vi "Apply Theme To TitleBar-Title.vi"(8 "Error In":errorcluster, 9 "Override Root With (Empty)":string, 10 "Title Ref":refnum<vi>, 11 "ini Theme in":refnum<class "ini Theme.lvclass">) -> (0 "Error Out":errorcluster, 3 "ini Theme out":refnum<class "ini Theme.lvclass">)   [LabVIEW 2021, in "Appearance Actor.lvlib" / "ini Theme.lvclass"]
uses:
  ini Theme.lvclass
  Generic Theme/API/Typedefs/Theme Entry--enum.ctl
  ini Theme.lvclass/ini Theme.ctl
  fa3b262b-9dee-4a2a-a40e-e8b24c2842d1.vi
  e580e7d3-37e0-4797-b7d4-6ea3cff1905c.vi
  b8bb2fda-9813-45b3-b864-ea548737c1bf.vi
  b36eaa81-33c9-40cb-a7ae-b56a33b86463.vi
  de97227f-fe4a-4e4e-bc85-f47ccb7673e6.vi
  5e2e6f35-8fd1-4567-afd0-e7bdc9ba1b23.vi
  7a2ed2a5-f796-4ddb-af4e-0a1f18797397.vi
  c737fe2c-22ae-4e1e-9e67-9ef794ffab69.vi
  <vilib>/Utility/config.llb/Read Key (U32).vi
  <vilib>/Utility/config.llb/Read Key (String).vi
  <vilib>/Utility/config.llb/NI_LVConfig.lvlib
  Generic Theme/Generic Theme.lvclass
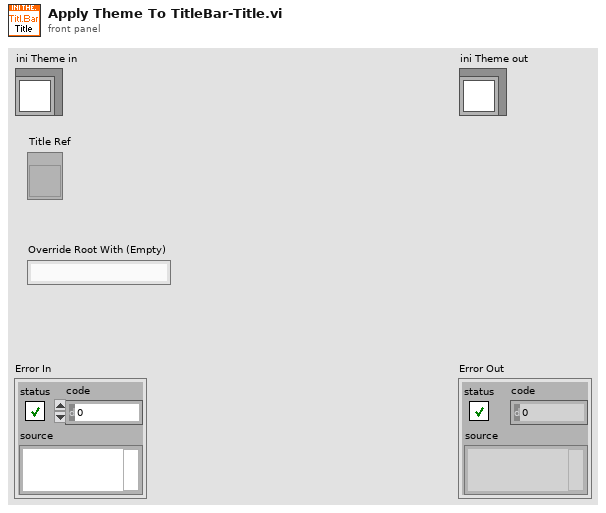
[diagram p1: front panel]
types:
  T1 = typedef "Appearance Actor.lvlib/Generic Theme.lvclass/Theme Entry--enum.ctl" = enum16{"None", "TitleBar.Pane.Color", "TitleBar.Splitter.FillColor", "TitleBar.Splitter.OutlineColor", "TitleBar.Title.Font.Color", "TitleBar.Title.Font.Family", "TitleBar.Title.Font.Size", "TitleBar.Title.Font.Style"}
  T2 = typedef "NI_LVConfig.lvlib/Config Data RefNum.ctl" = refnum<k1>
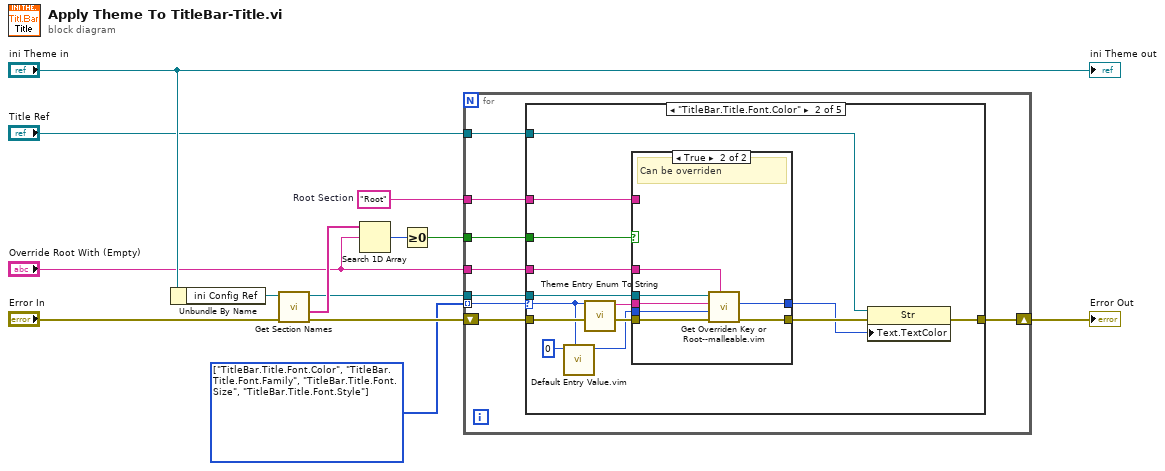
[diagram p0: block diagram]
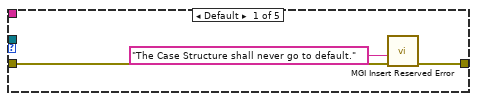
[diagram p2: hidden frame]
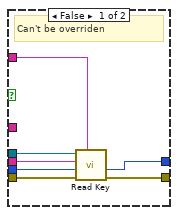
[diagram p3: hidden frame]
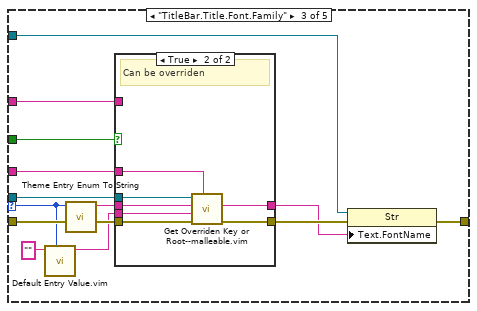
[diagram p4: hidden frame]
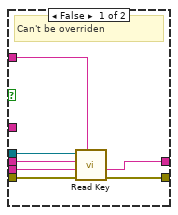
[diagram p5: hidden frame]
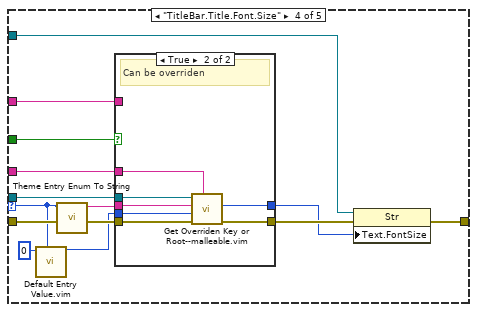
[diagram p6: hidden frame]
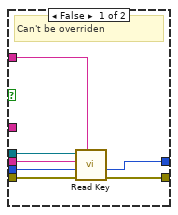
[diagram p7: hidden frame]
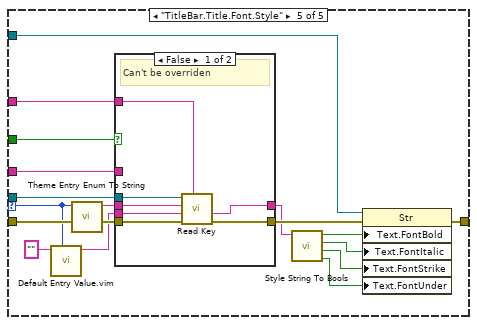
[diagram p8: hidden frame]
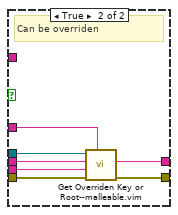
[diagram p9: hidden frame]
diagram:
  w1 = T1[] [enum."TitleBar.Title.Font.Color", enum."TitleBar.Title.Font.Family", enum."TitleBar.Title.Font.Size", enum."TitleBar.Title.Font.Style"] items=["None", "TitleBar.Pane.Color", "TitleBar.Splitter.FillColor", "TitleBar.Splitter.OutlineColor", "TitleBar.Title.Font.Color", "TitleBar.Title.Font.Family", "TitleBar.Title.Font.Size", "TitleBar.Title.Font.Style"] ("Array")
  w3 = "Root"  # Root Section
  n1 = Unbundle By Name("ini Theme in") -> ("ini Config Ref"=w13:T2)
  n2 = call <vilib>:"Get Section Names.vi"("error in (no error)"="Error In", "refnum"=w13) -> ("error out"=w10:errorcluster, "section names"=w12:string[], "refnum out"=w4:T2)  [unwired: 7 in]
  n3 = Search 1D Array(1D array=w12, element="Override Root With (Empty)") -> (index of element=w11:i32)  [unwired: 1 in]
  n4 = Greater Or Equal To 0?(x=w11) -> (x >= 0?=w5:bool)
  n5 = for {
    shift-right: [w15] -> w8
    shift-left: w10 -> [w21]
    tunnel: "Override Root With (Empty)" -> [w20]
    tunnel: w5 -> [w19]
    tunnel: w4 -> [w18]
    tunnel: w3 -> [w17]
    tunnel: w1 -> [w16] mode=indexing
    tunnel: "Title Ref" -> [w14]
    n6 = case shown="\"TitleBar.Title.Font.Color\"" w16 {
      selector: w16 -> [_ w27 w54 w82 w112]
      tunnel: w21 -> [w23 w37 w64 w91 w122]
      tunnel: w20 -> [_ w35 w62 w89 w120]
      tunnel: w19 -> [_ w34 w61 w88 w119]
      tunnel: w18 -> [_ w33 w60 w87 w118]
      tunnel: w17 -> [_ w32 w59 w86 w117]
      tunnel: [w22 w31 w58 w85 w116] -> w15
      tunnel: w14 -> [_ w30 w57 w84 w115]
      frame Default {
        n7 = call <userlib>:"MGI Insert Reserved Error.vi"("Error In"=w23, "Error Description"="The Case Structure shall never go to default.") -> ("Error Out"=w22:errorcluster)  [unwired: 9 in]
      }
      frame "TitleBar.Title.Font.Color" {
        n8 = call "Default Entry Value.vim"("Root Theme Entry"=w27, "Data Type"=u32 0) -> ("Default Value"=w26:u32)  [unwired: 9 in]
        n9 = call "Theme Entry Enum To String.vi"("Root Theme Entry"=w27) -> ("Root Theme Entry String"=w28:string)  [unwired: 10 in]
        n10 = case shown="True" w34 {
          tunnel: w37 -> [w44 w51]
          tunnel: [w43 w50] -> w36
          tunnel: w35 -> [_ w49]
          tunnel: w33 -> [w41 w48]
          tunnel: w32 -> [w42 _]
          tunnel: w28 -> [w40 w47]
          tunnel: w26 -> [w38 w46]
          tunnel: [w39 w45] -> w29
          frame False {
            # "Can't be overriden"
            n11 = call-poly <vilib>:"Read Key.vi"("section"=w42, "error in (no error)"=w44, "default value"=w38, "key"=w40, "refnum"=w41) -> ("error out"=w43:errorcluster, "value"=w39:u32)  [unwired: 3 in, 2 out]
          }
          frame True {
            # "Can be overriden"
            n12 = call "Get Overriden Key or Root--malleable.vim"("Override Root With"=w49, "Error In"=w51, "Default"=w46, "Key"=w47, "ini Ref In"=w48) -> ("Error Out"=w50:errorcluster, "Value"=w45:u32)  [unwired: 4 in, 1 out]
          }
        }
        n13 = property class="Str"(reference=w30, error in=w36, "Text.TextColor"=w29) -> (error out=w31:errorcluster)  [unwired: 1 out]
      }
      frame "TitleBar.Title.Font.Family" {
        n14 = call "Default Entry Value.vim"("Root Theme Entry"=w54, "Data Type"="") -> ("Default Value"=w53:string)  [unwired: 9 in]
        n15 = call "Theme Entry Enum To String.vi"("Root Theme Entry"=w54) -> ("Root Theme Entry String"=w55:string)  [unwired: 10 in]
        n16 = case shown="True" w61 {
          tunnel: w64 -> [w71 w78]
          tunnel: [w70 w77] -> w63
          tunnel: w62 -> [_ w76]
          tunnel: w60 -> [w68 w75]
          tunnel: w59 -> [w69 _]
          tunnel: w55 -> [w67 w74]
          tunnel: w53 -> [w65 w73]
          tunnel: [w66 w72] -> w56
          frame False {
            # "Can't be overriden"
            n17 = call-poly <vilib>:"Read Key.vi"("section"=w69, "error in (no error)"=w71, "default value"=w65, "key"=w67, "refnum"=w68) -> ("error out"=w70:errorcluster, "value"=w66:string)  [unwired: 3 in, 2 out]
          }
          frame True {
            # "Can be overriden"
            n18 = call "Get Overriden Key or Root--malleable.vim"("Override Root With"=w76, "Error In"=w78, "Default"=w73, "Key"=w74, "ini Ref In"=w75) -> ("Error Out"=w77:errorcluster, "Value"=w72:string)  [unwired: 4 in, 1 out]
          }
        }
        n19 = property class="Str"(reference=w57, error in=w63, "Text.FontName"=w56) -> (error out=w58:errorcluster)  [unwired: 1 out]
      }
      frame "TitleBar.Title.Font.Size" {
        n20 = call "Default Entry Value.vim"("Root Theme Entry"=w82, "Data Type"=u32 0) -> ("Default Value"=w80:u32)  [unwired: 9 in]
        n21 = call "Theme Entry Enum To String.vi"("Root Theme Entry"=w82) -> ("Root Theme Entry String"=w81:string)  [unwired: 10 in]
        n22 = case shown="True" w88 {
          tunnel: w91 -> [w98 w105]
          tunnel: [w97 w104] -> w90
          tunnel: w89 -> [_ w103]
          tunnel: w87 -> [w95 w102]
          tunnel: w86 -> [w96 _]
          tunnel: w81 -> [w94 w101]
          tunnel: w80 -> [w92 w100]
          tunnel: [w93 w99] -> w83
          frame False {
            # "Can't be overriden"
            n23 = call-poly <vilib>:"Read Key.vi"("section"=w96, "error in (no error)"=w98, "default value"=w92, "key"=w94, "refnum"=w95) -> ("error out"=w97:errorcluster, "value"=w93:u32)  [unwired: 3 in, 2 out]
          }
          frame True {
            # "Can be overriden"
            n24 = call "Get Overriden Key or Root--malleable.vim"("Override Root With"=w103, "Error In"=w105, "Default"=w100, "Key"=w101, "ini Ref In"=w102) -> ("Error Out"=w104:errorcluster, "Value"=w99:u32)  [unwired: 4 in, 1 out]
          }
        }
        n25 = property class="Str"(reference=w84, error in=w90, "Text.FontSize"=w83) -> (error out=w85:errorcluster)  [unwired: 1 out]
      }
      frame "TitleBar.Title.Font.Style" {
        n26 = call "Default Entry Value.vim"("Root Theme Entry"=w112, "Data Type"="" ("Default")) -> ("Default Value"=w114:string)  [unwired: 9 in]
        n27 = call "Theme Entry Enum To String.vi"("Root Theme Entry"=w112) -> ("Root Theme Entry String"=w111:string)  [unwired: 10 in]
        n28 = case shown="False" w119 {
          tunnel: w122 -> [w129 w136]
          tunnel: [w128 w135] -> w121
          tunnel: w120 -> [_ w134]
          tunnel: w118 -> [w126 w133]
          tunnel: w117 -> [w127 _]
          tunnel: w111 -> [w125 w132]
          tunnel: w114 -> [w123 w131]
          tunnel: [w124 w130] -> w109
          frame False {
            # "Can't be overriden"
            n29 = call-poly <vilib>:"Read Key.vi"("section"=w127, "error in (no error)"=w129, "default value"=w123, "key"=w125, "refnum"=w126) -> ("error out"=w128:errorcluster, "value"=w124:string)  [unwired: 3 in, 2 out]
          }
          frame True {
            # "Can be overriden"
            n30 = call "Get Overriden Key or Root--malleable.vim"("Override Root With"=w134, "Error In"=w136, "Default"=w131, "Key"=w132, "ini Ref In"=w133) -> ("Error Out"=w135:errorcluster, "Value"=w130:string)  [unwired: 4 in, 1 out]
          }
        }
        n31 = call "Style String To Bools.vi"("Style String"=w109) -> ("Underlined"=w106:bool, "Strikeout"=w107:bool, "Italic"=w108:bool, "Bold"=w110:bool)  [unwired: 7 in]
        n32 = property class="Str"(reference=w115, error in=w121, "Text.FontBold"=w110, "Text.FontItalic"=w108, "Text.FontStrike"=w107, "Text.FontUnder"=w106) -> (error out=w116:errorcluster)  [unwired: 1 out]
      }
    }
  }
  "Error Out" <- w8
  "ini Theme out" <- "ini Theme in"
